vi "GetIOReadStatusMerge.vi"   [LabVIEW 2020]
doc: "Reports the status of reading I/O data from the I/O items."
uses:
  <vilib>/eio/EIOGrowableMethodNode/genericMethod/EIOGrowableMethodNode.xnode
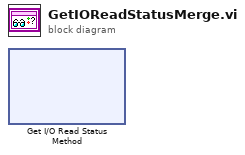
[diagram p0: block diagram]
diagram:
  n1 = xnode "Get I/O Read Status Method"() -> ()  [unwired: 1 in, 3 out]
